vi "BotSpeak_FindBot.vi"(3 "String To Send":string, 4 "Reset?":bool, 5 "Bot Settings":T2) -> (0 "Reply":string, 1 "String Sent":string, 2 "Connection":T1)   [LabVIEW 2012]
uses:
  <userlib>/BotSpeak/VIs/SubVIs/CommState.ctl
  <userlib>/BotSpeak/VIs/Direct/BotSpeak_Control.ctl
  <userlib>/BotSpeak/VIs/SubVIs/BotSpeak_Globals.vi
panel:
  out "Bot#":i32
  out "Bots":T1[](array[typedef])
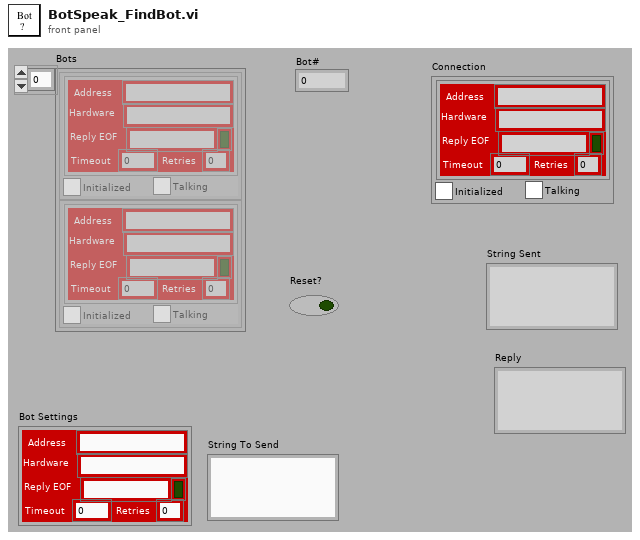
[diagram p1: front panel]
types:
  T1 = typedef "CommState.ctl" = cluster{"Bot Settings":T2, "Initialized":bool, "Talking":bool}
  T2 = typedef "BotSpeak_Control.ctl" = cluster{"Address":string, "Reply EOF":string, "Hardware":string, "Retries":i8, "Timeout":i32, "Open?":bool}
  T3 = typedef "BotSpeak_Control.ctl" = cluster{"Address":string, "Reply EOF":string, "Hardware":string, "Retries":i8, "Timeout":i32}
  T4 = cluster{"Last Bot":T2, "Abort?":bool, "Abort?":bool}
  T5 = cluster{"Reply":string, "Reply":string, "Reply":string}
  T6 = cluster{"Sent":string, "reply":string, "Botspeak Script":string}[]
  T7 = cluster{"Reply":string, "Reply":string, "Reply":string}[]
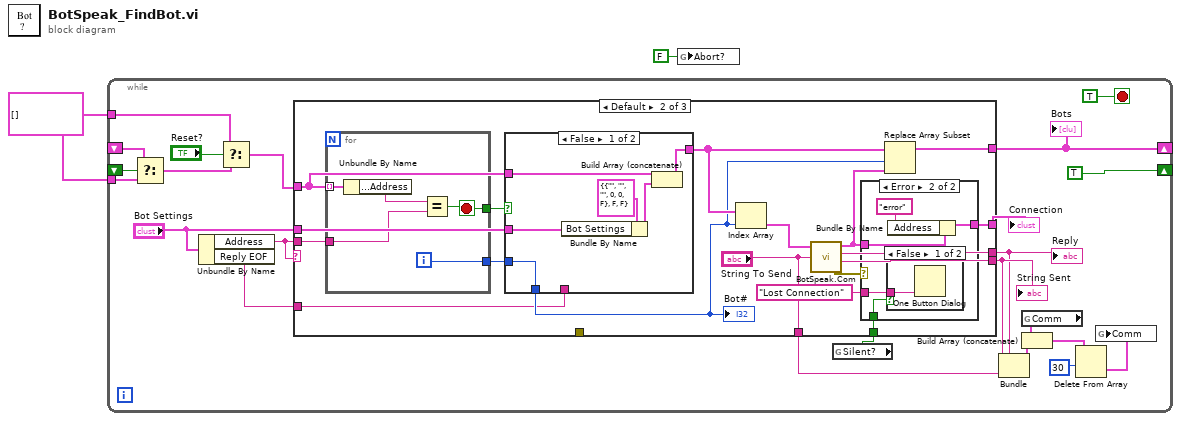
[diagram p0: block diagram]
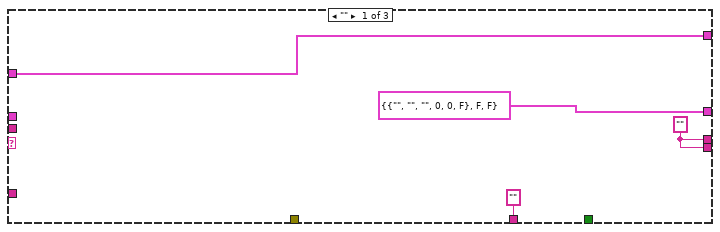
[diagram p2: hidden frame]
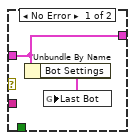
[diagram p3: hidden frame]
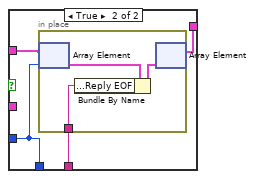
[diagram p5: hidden frame]
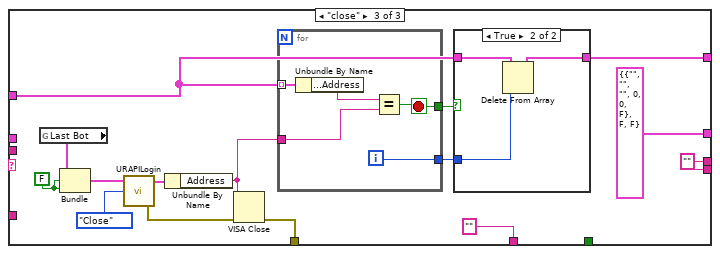
[diagram p6: hidden frame]
diagram:
  w1 = T1[] [] ("Bots")
  n1 = while {
    shift-right: [TRUE] -> _
    shift-left: _ -> [w14]
    shift-right: [w23] -> _
    shift-left: _ -> [w13]
    tunnel: w1 -> [w9]
    tunnel: w1 -> [w12]
    stop <- TRUE stop-if-true
    n2 = Select(t=w13, s=w14, f=w12) -> (s? t:f=w10:T1[])
    n3 = Unbundle By Name("Bot Settings") -> ("Address"=w20:string, "Reply EOF"=w15:string)
    n4 = Select(t=w9, s="Reset?", f=w10) -> (s? t:f=w8:T1[])
    n5 = global read "BotSpeak_Globals.vi" "Silent?"() -> (w3:bool)
    n6 = case shown="Default" w20 {
      tunnel: w8 -> [w29 w37 w83]
      tunnel: [w27 w43 w87] -> w16
      tunnel: [w27 w42 w87] -> w17
      tunnel: [w29 w40 w82] -> w23
      tunnel: [T1 {"Bot Settings"={"Address"="", "Reply EOF"="", "Hardware"="", "Retries"=0, "Timeout"=0, "Open?"=FALSE}, "Initialized"=FALSE, "Talking"=FALSE} ("Connections out") w34 T1 {"Bot Settings"={"Address"="", "Reply EOF"="", "Hardware"="", "Retries"=0, "Timeout"=0, "Open?"=FALSE}, "Initialized"=FALSE, "Talking"=FALSE} ("Connection out")] -> w22
      tunnel: "Bot Settings" -> [_ w39 _]
      tunnel: w20 -> [_ w38 _]
      tunnel: w15 -> [_ w32 _]
      tunnel: [_ _ w88] -> _
      tunnel: ["" ("Reply") "String To Send" "" ("Reply")] -> w7
      tunnel: w3 -> [_ w30 _]
      frame "" {
        w27 = "" ("Reply")
      }
      frame Default {
        n7 = for {
          tunnel: w37 -> [w73] mode=indexing
          tunnel: [w71] -> w47
          tunnel: [w69] -> w46
          tunnel: w38 -> [w70]
          i -> [w69]
          stop <- w71 stop-if-true
          n8 = Unbundle By Name(w73) -> ("Bot Settings.Address"=w72:string)
          n9 = Equal?(x=w72, y=w70) -> (x = y?=w71:bool)
        }
        n10 = case shown="False" w47 {
          tunnel: w37 -> [w61 w65]
          tunnel: [w60 w63] -> w45
          tunnel: w39 -> [w56 _]
          tunnel: w46 -> [w58 w64]
          tunnel: [w58 w64] -> w44
          tunnel: w32 -> [_ w62]
          frame False {
            n11 = Bundle By Name(cluster=T1 {"Bot Settings"={"Address"="", "Reply EOF"="", "Hardware"="", "Retries"=0, "Timeout"=0, "Open?"=FALSE}, "Initialized"=FALSE, "Talking"=FALSE} ("Connections In"), "Bot Settings"=w56) -> (w59:T1)
            n12 = Build Array (concatenate)(w61, w59) -> (w60:T1[])
          }
          frame True {
            n13 = in-place {
              in-place-border: w62 -> [w66]
              n14 = in-place-array #1(w65, w64) -> (w68:T1)
              n15 = Bundle By Name(cluster=w68, "Bot Settings.Reply EOF"=w66) -> (w67:T1)
              n16 = in-place-array #1(w67) -> (w63:T1[])  [unwired: 1 out]
            }
          }
        }
        "Bot#" <- w44
        n17 = Index Array(array=w45, index=w44) -> (element=w41:T1)
        n18 = call <userlib>:"BotSpeak.Com.vi"("To Send"="String To Send", "Bot Settings in"=w41) -> ("error out"=w36:errorcluster, "Sent"=w42:string, "Reply"=w43:string, "Bot Settings out"=w33:T2)  [unwired: 1 in]
        n19 = case shown="Error" w36 {
          tunnel: "Lost Connection" -> [_ w54]
          tunnel: [w48 w52] -> w34
          tunnel: w33 -> [w48 w53]
          tunnel: w30 -> [_ w50]
          frame No Error {
            n20 = Unbundle By Name(w48) -> ("Bot Settings"=w49:T3)
            n21 = global write "BotSpeak_Globals.vi" "Last Bot"(w49) -> ()
          }
          frame Error {
            n22 = case shown="False" w50 {
              tunnel: w54 -> [w55 _]
              frame False {
                n23 = One Button Dialog(message=w55) -> ()  [unwired: 1 in, 1 out]
              }
              frame True {
              }
            }
            n24 = Bundle By Name(cluster=w53, "Address"="error" ("Bot Settings.Address")) -> (w52:T2)
          }
        }
        n25 = Replace Array Subset(array=w45, new element=w33, index=w44) -> (w40:T1[])
      }
      frame "close" {
        w79 = FALSE ("Abort?")
        w87 = "" ("Reply")
        n26 = global read "BotSpeak_Globals.vi" "Last Bot"() -> (w80:T2)
        n27 = Bundle("Last Bot"=w80, "Abort?"=w79, "Abort?"=w79) -> (w77:T4)  [unwired: 1 in]
        n28 = call <userlib>:"URAPILogin.vi"("Task"=enum16{"Init", "Close"}."Close", "Bot Settings in"=w77) -> ("error out"=w75:errorcluster, "Bot Settings out"=w76:T2)  [unwired: 1 in]
        n29 = Unbundle By Name(w76) -> ("Address"=w85:string)
        n30 = VISA Close(VISA resource name=w85, error in (no error)=w75) -> (error out=w88:errorcluster)
        n31 = for {
          tunnel: w83 -> [w97] mode=indexing
          tunnel: [w95] -> w84
          tunnel: [w93] -> w81
          tunnel: w85 -> [w94]
          i -> [w93]
          stop <- w95 stop-if-true
          n32 = Unbundle By Name(w97) -> ("Bot Settings.Address"=w96:string)
          n33 = Equal?(x=w96, y=w94) -> (x = y?=w95:bool)
        }
        n34 = case shown="True" w84 {
          tunnel: w83 -> [w89 w92]
          tunnel: [w89 w91] -> w82
          tunnel: w81 -> [_ w90]
          frame False {
          }
          frame True {
            n35 = Delete From Array(array=w92, index=w90) -> (array with subset deleted=w91:T1[])  [unwired: 1 in, 1 out]
          }
        }
      }
    }
    "Bots" <- w23
    "String Sent" <- w17
    "Connection" <- w22
    "Reply" <- w16
    n36 = Bundle("Reply"=w17, "Reply"=w16, "Reply"=w7) -> (w18:T5)  [unwired: 1 in]
    n37 = global read "BotSpeak_Globals.vi" "Comm"() -> (w19:T6)
    n38 = Build Array (concatenate)(w19, w18) -> (w6:T7)
    n39 = Delete From Array(array=w6, length=30) -> (deleted portion=w5:T7)  [unwired: 1 in, 1 out]
    n40 = global write "BotSpeak_Globals.vi" "Comm"(w5) -> ()
  }
  n41 = global write "BotSpeak_Globals.vi" "Abort?"(FALSE ("Abort?")) -> ()
